vi "Initialize.vi"(8 "Error In":errorcluster, 11 "Parser In":refnum<class "Parser.lvclass">) -> (0 "Error Out":errorcluster, 3 "Parser Out":refnum<class "Parser.lvclass">)   [LabVIEW 2018, in "Toolkit.lvlib" / "Parser.lvclass"]
uses:
  Parser.lvclass
  Parser.lvclass/Parser.ctl
  Nodes/NonTerminal/NonTerminal.lvclass
  Nodes/Root/Root.lvclass
  D:/Users/cfield/Code/Field R&D Services/Labstache/src/Toolkit/Low-Level/Nodes/NonTerminal/NonTerminal.lvclass
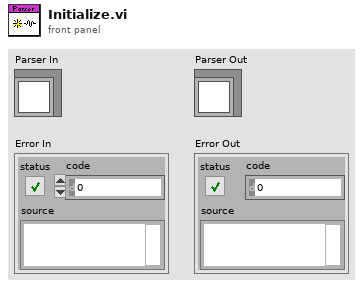
[diagram p1: front panel]
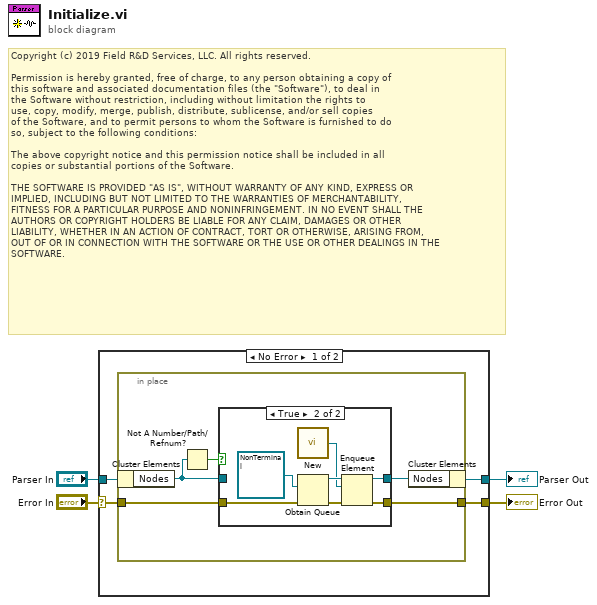
[diagram p0: block diagram]
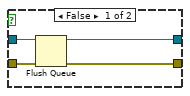
[diagram p2: hidden frame]
diagram:
  # "Copyright (c) 2019 Field R&D Services, LLC. All rights reserved.\n\nPermission is hereby granted, free of charge, to any person obtaining a copy of\nthis software and associated documentation files (the \"Software\"), to deal in\nthe Software without restriction, including without limitation the rights to\nuse, copy, modify, merge, publish, distribute, sublicense, and/or sell copies\nof the Software, and to permit persons to whom the Software is furnished to do\nso, subject to the following conditions:\n\nThe above copyright notice and this permission notice shall be included in all\ncopies or substantial portions of the Software.\n\nTHE SOFTWARE IS PROVIDED \"AS IS\", WITHOUT WARRANTY OF ANY KIND, EXPRESS OR\nIMPLIED, INCLUDING BUT NOT LIMITED TO THE WARRANTIES OF MERCHANTABILITY,\nFITNESS FOR A PARTICULAR PURPOSE AND NONINFRINGEMENT. IN NO EVENT SHALL THE\nAUTHORS OR COPYRIGHT HOLDERS BE LIABLE FOR ANY CLAIM, DAMAGES OR OTHER\nLIABILITY, WHETHER IN AN ACTION OF CONTRACT, TORT OR OTHERWISE, ARISING FROM,\nOUT OF OR IN CONNECTION WITH THE SOFTWARE OR THE USE OR OTHER DEALINGS IN THE\nSOFTWARE."
  n1 = case shown="No Error" "Error In" {
    selector: "Error In" -> [w8 w26]
    tunnel: [w6 w26] -> w4
    tunnel: "Parser In" -> [w7 w25]
    tunnel: [w5 w25] -> w1
    frame No Error {
      n2 = in-place {
        in-place-border: w8 -> [w13]
        in-place-border: [w9] -> w6
        n3 = in-place-cluster #1(w7) -> ("Nodes"=w10:refnum<queue>)
        n4 = Not A Number/Path/Refnum?(number/path/refnum=w10) -> (NaN/Path/Refnum?=w12:bool)
        n5 = case shown="True" w12 {
          tunnel: w13 -> [w14 w20]
          tunnel: [w16 w19] -> w11
          tunnel: w10 -> [w17 _]
          tunnel: [w15 w18] -> w9
          frame False {
            n6 = Flush Queue(queue=w17, error in (no error)=w14) -> (queue out=w16:refnum<queue>, error out=w15:errorcluster)  [unwired: 1 out]
          }
          frame True {
            n7 = call "New.vi"() -> ("Root"=w21:refnum<class "Root.lvclass">)
            n8 = Obtain Queue(element data type=refnum<class "NonTerminal.lvclass"> refnum ("Toolkit.lvlib:Nodes.lvlib:NonTerminal.lvclass"), error in (no error)=w20) -> (queue out=w23:refnum<queue>, error out=w22:errorcluster)  [unwired: 3 in, 1 out]
            n9 = Enqueue Element(queue=w23, element=w21, error in (no error)=w22) -> (queue out=w19:refnum<queue>, error out=w18:errorcluster)  [unwired: 1 in, 1 out]
          }
        }
        n10 = in-place-cluster #1("Nodes"=w11) -> (w5:refnum<class "Parser.lvclass">)
      }
    }
    frame Error {
    }
  }
  "Parser Out" <- w1
  "Error Out" <- w4
